vi "execute.vi"(8 "error in (no error)":errorcluster, 10 "Context in":refnum<class "Context.lvclass">, 11 "TestHardpointCommand in":refnum<class "TestHardpointCommand.lvclass">) -> (0 "error out":errorcluster, 2 "Context out":refnum<class "Context.lvclass">, 3 "TestHardpointCommand out":refnum<class "TestHardpointCommand.lvclass">)   [LabVIEW 2016, in "TestHardpointCommand.lvclass"]
uses:
  TestHardpointCommand.lvclass
  Context/Context.lvclass
  TestHardpointCommand.lvclass/TestHardpointCommand.ctl
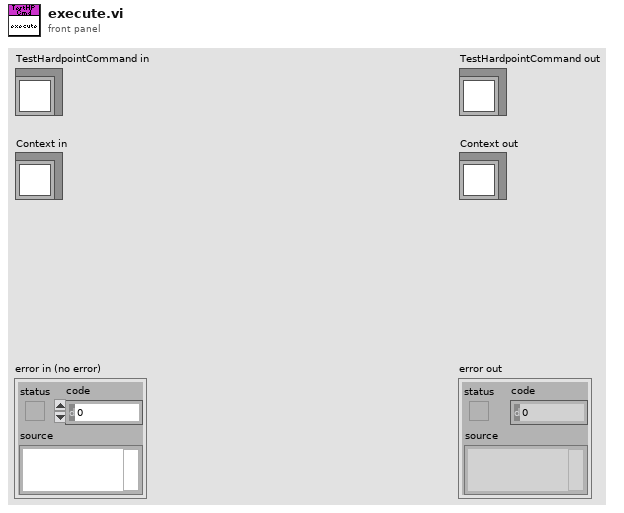
[diagram p1: front panel]
types:
  T1 = typedef "M1M3SupportTopics.lvlib/CommandTestHardpoint.ctl" = cluster{"CommandId":T2, "ActuatorId":i32}
  T2 = typedef "M1M3SupportTopics.lvlib/CommandId.ctl" = i32
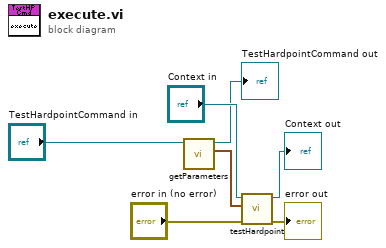
[diagram p0: block diagram]
diagram:
  n1 = call "getParameters.vi"("TestHardpointCommand in"="TestHardpointCommand in") -> ("Parameters"=w1:T1, "TestHardpointCommand out"=→"TestHardpointCommand out":refnum<class "TestHardpointCommand.lvclass">)  [unwired: 9 in]
  n2 = call-dynamic "testHardpoint.vi"("error in (no error)"="error in (no error)", "Parameters"=w1, "Context in"="Context in") -> ("error out"=→"error out":errorcluster, "Context out"=→"Context out":refnum<class "Context.lvclass">)  [unwired: 7 in]
